vi "1D experiment mouse.vi"() -> ()   [LabVIEW 2011]
uses:
  <vilib>/Platform/TimedLoop/XDataNode/timing_clust.ctl
  <vilib>/Platform/TimedLoop/XDataNode/nitl_modes.ctl
  <vilib>/Platform/TimedLoop/XDataNode/wakeup.ctl
  <vilib>/Utility/inputDevices.llb/closeMouse.vi
  <vilib>/Utility/cursorutil.llb/Set Cursor (Cursor ID).vi
  <vilib>/Utility/inputDevices.llb/mouseAcquire.vi
  <vilib>/Utility/file.llb/Write To Spreadsheet File (DBL).vi
  <vilib>/Utility/file.llb/Write To Spreadsheet File (I64).vi
  <vilib>/Platform/TimedLoop/XDataNode/XDataNode.xnode
  <vilib>/Platform/TimedLoop/XDataNode/XDNodeRunTimeDep.lvlib
  User32.dll
panel:
  out "initial time":u32
  out "1D Experiment":cluster{"Y":dbl[], "Y":dbl[]}[](graph)
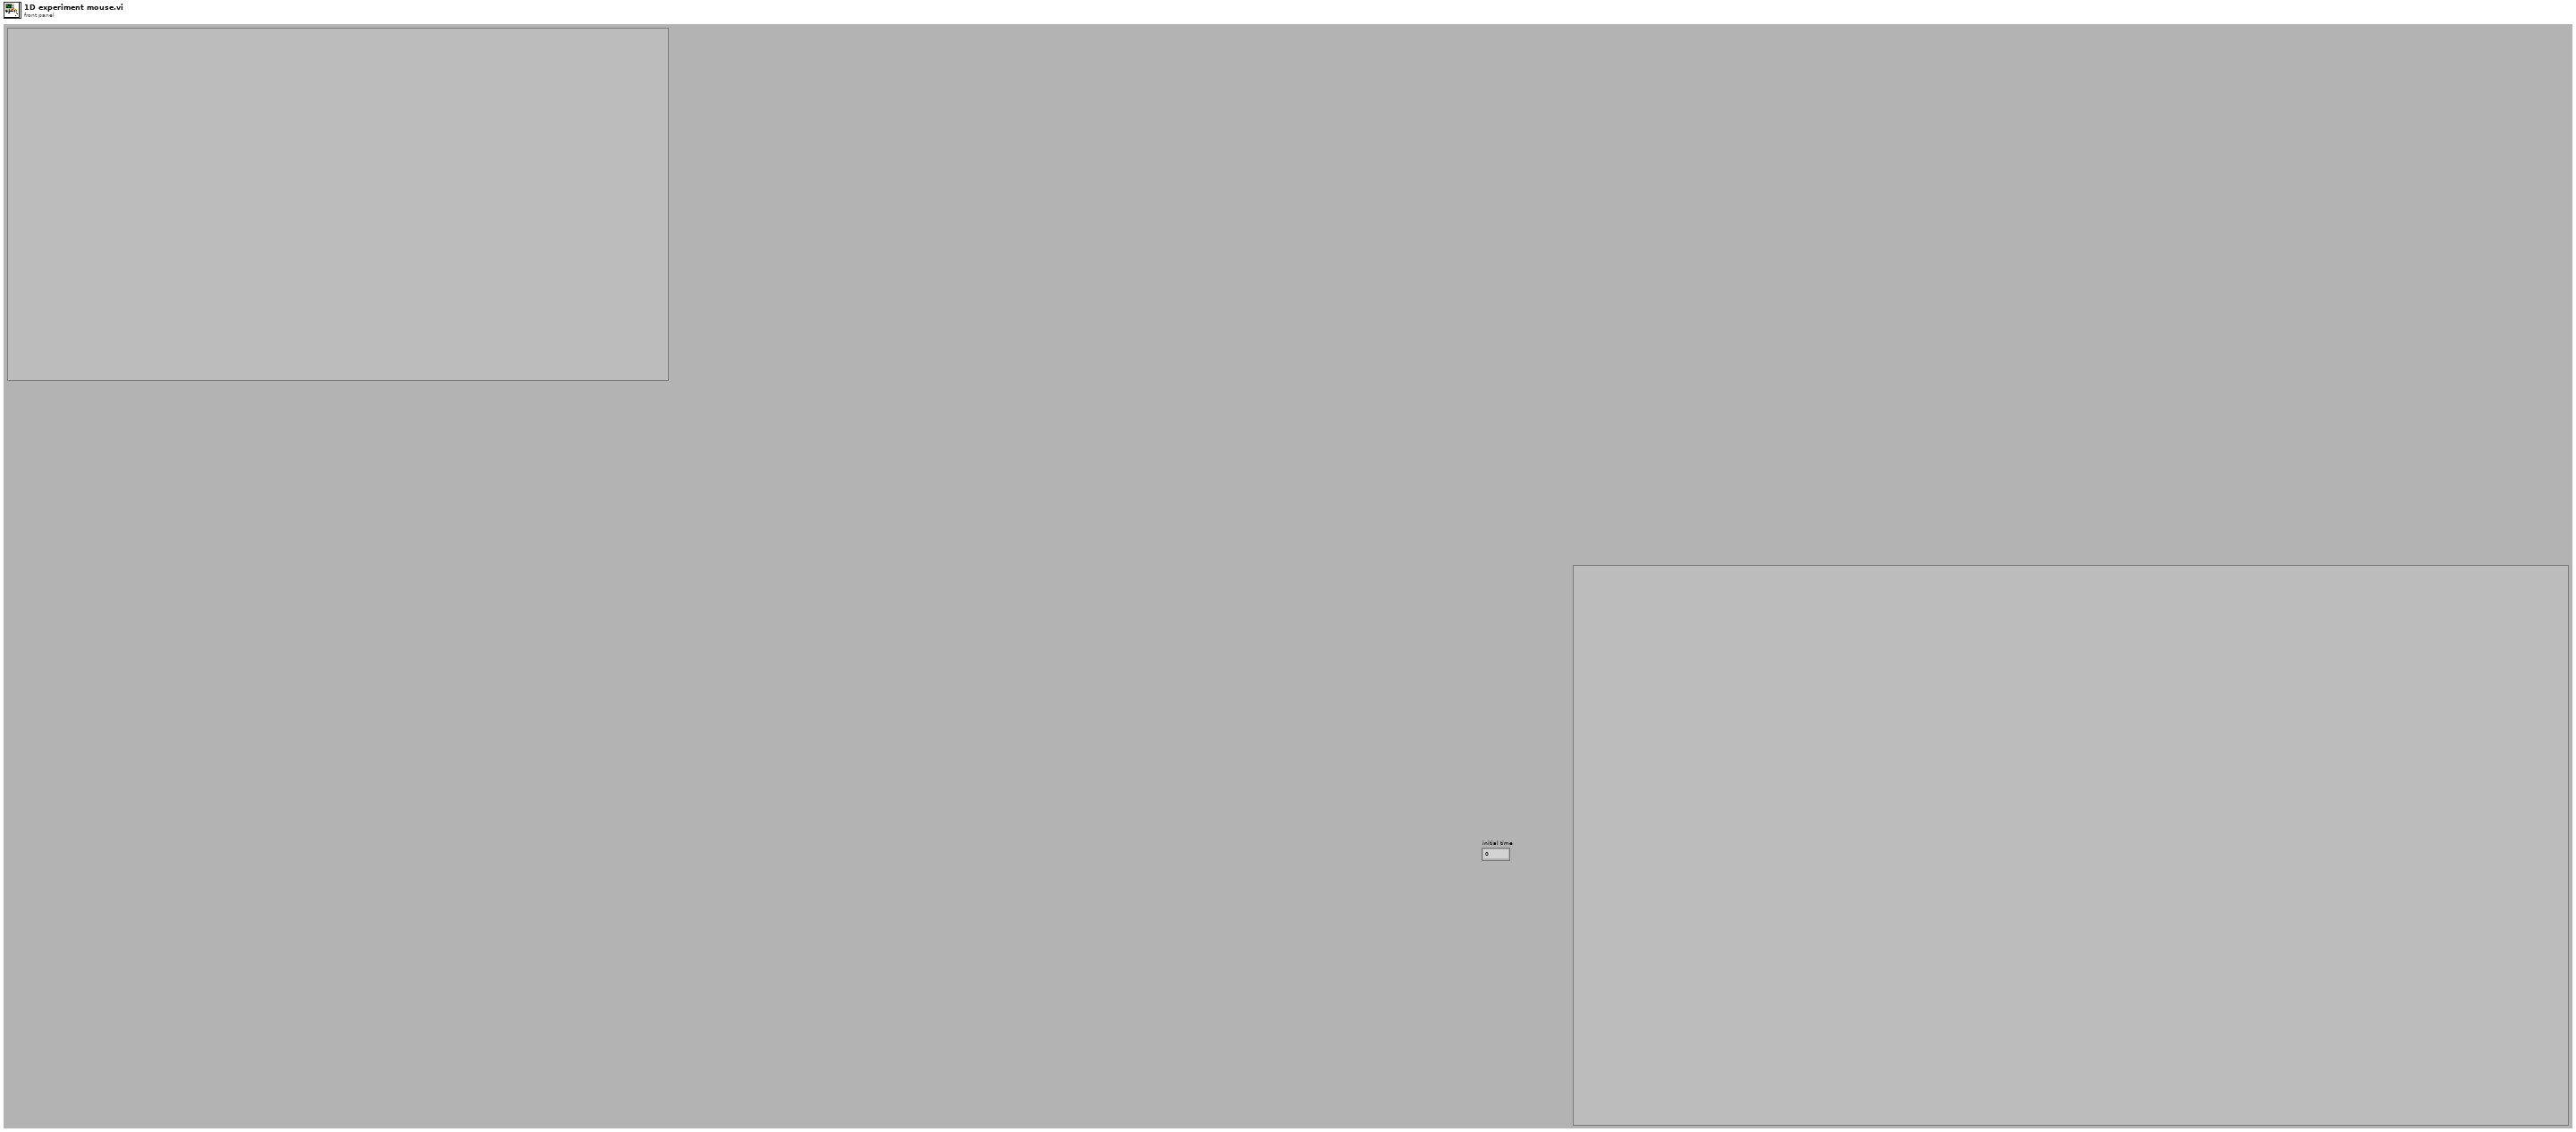
[diagram p1: front panel]
types:
  T1 = enum16{"open", "replace", "create", "open or create", "replace or create", "replace or create with confirmation"}
  T2 = typedef "XDNodeRunTimeDep.lvlib/timing_clust.ctl" = cluster{"Expected End [f-1]":u64, "Actual End [f-1]":u64, "Finished Late? [f-1]":bool, "Expected End [i-1]":u64, "Actual End [i-1]":u64, "Finished Late? [i-1]":bool, "Expected Start [i]":u64, "Actual Start [i]":u64, "Expected Start [f]":u64, "Actual Start [f]":u64, "Source Name":string, "Structure Name":string, "Period":i64, "Deadline":i64, "Offset":i64, "Start":i64, "Priority":i32, "Timeout":i32, "Mode":T3, "Wakeup Reason":T4, "Error":errorcluster, "Source Type":string, "Secondary Source Type":string, "Global End Time":u64, "Global Start Time":u64, "Frame Duration":u64, "Iteration Duration":u64, "Assigned CPU":i32, "I/O Scan Engine Mode":u32}
  T3 = typedef "XDNodeRunTimeDep.lvlib/nitl_modes.ctl" = enum32{"No Change", "Process missed periods, maintain original phase", "Discard missed periods, maintain original phase", "Process missed periods, ignore original phase", "Discard missed periods, ignore original phase"}
  T4 = typedef "XDNodeRunTimeDep.lvlib/wakeup.ctl" = enum32{"Normal", "Aborted", "Asynchronous wakeup", "Timing source error", "Timed loop error", "Timeout"}
  T5 = cluster{"Radius":dbl, "x0":dbl, "y0":dbl, "D":dbl, bool}
  T6 = typedef "LVAllMonitorsDisplayTypeDef.ctl" = cluster{"Bounds":cluster{"Left":i16, "Top":i16, "Right":i16, "Bottom":i16}, "Depth":i16}[]
  T7 = cluster{"Bounds":cluster{"Left":i16, "Top":i16, "Right":i16, "Bottom":i16}, "Depth":i16}
  T8 = cluster{"Left":i16, "Top":i16, "Right":i16, "Bottom":i16}
  T9 = cluster{"Horizontal":i32, "Vertical":i32, "Scrolling":i32}
  T10 = cluster{"button 1":bool, "button 2":bool, "button 3":bool, "button 4":bool}
  T11 = typedef "LVPoint32TypeDef.ctl" = cluster{"Horizontal":i32, "Vertical":i32}
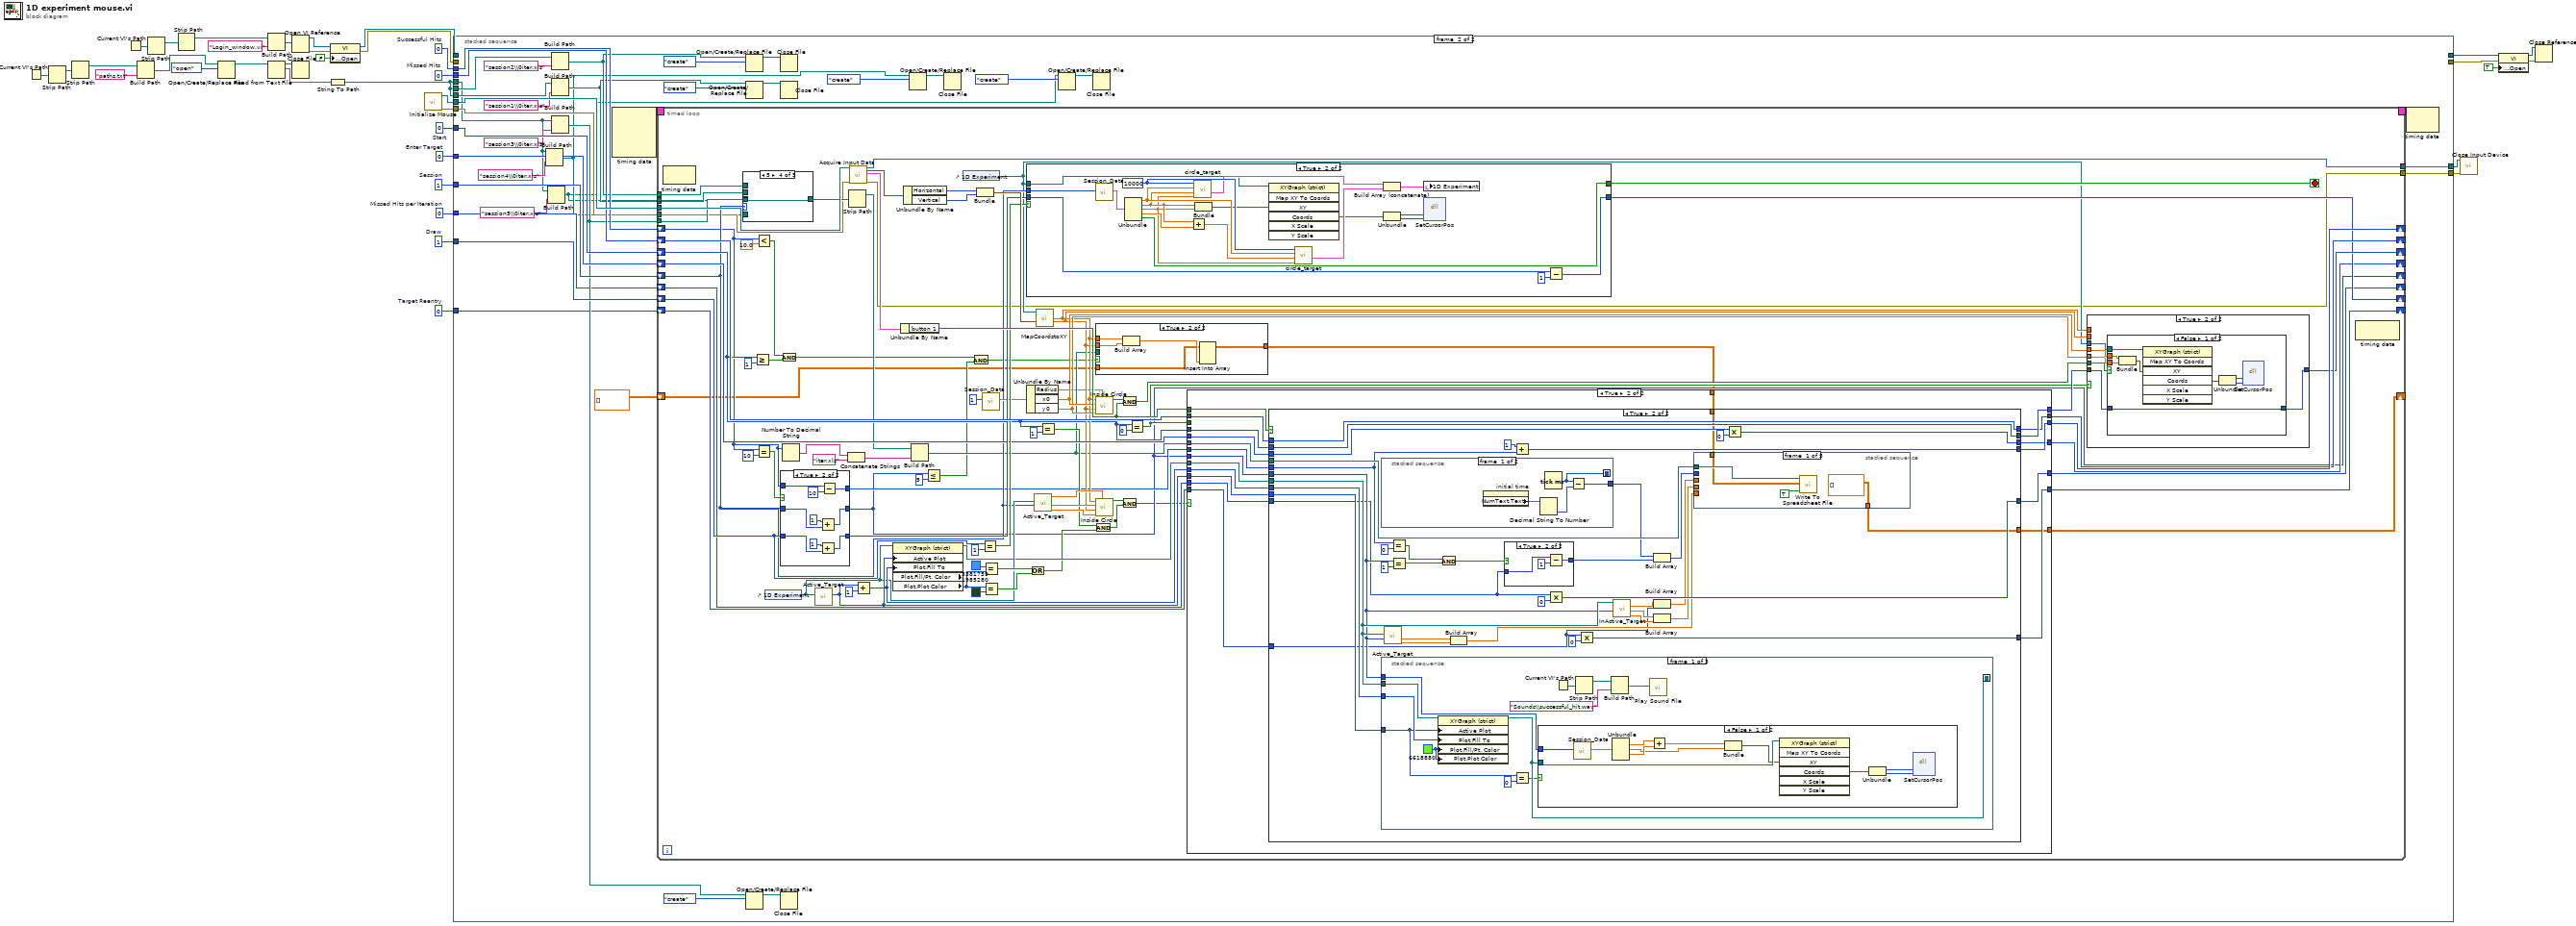
[diagram p0: block diagram]
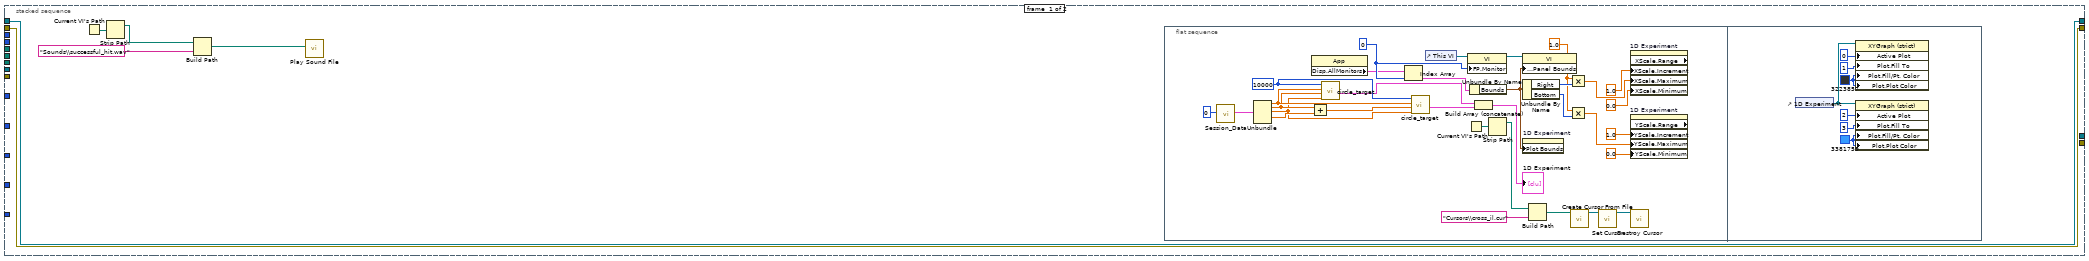
[diagram p2: hidden frame]
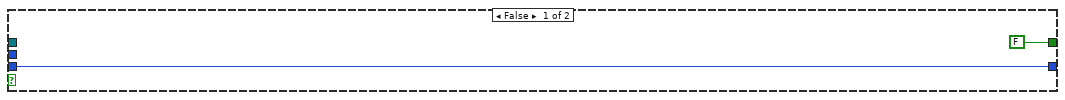
[diagram p8: hidden frame]
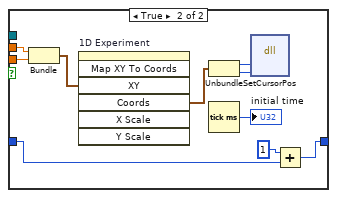
[diagram p10: hidden frame]
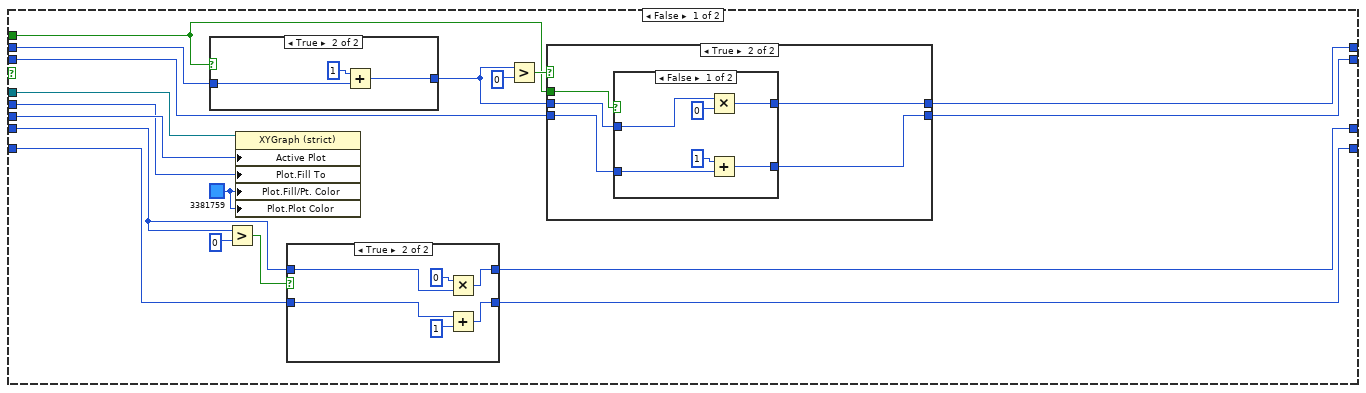
[diagram p13: hidden frame]
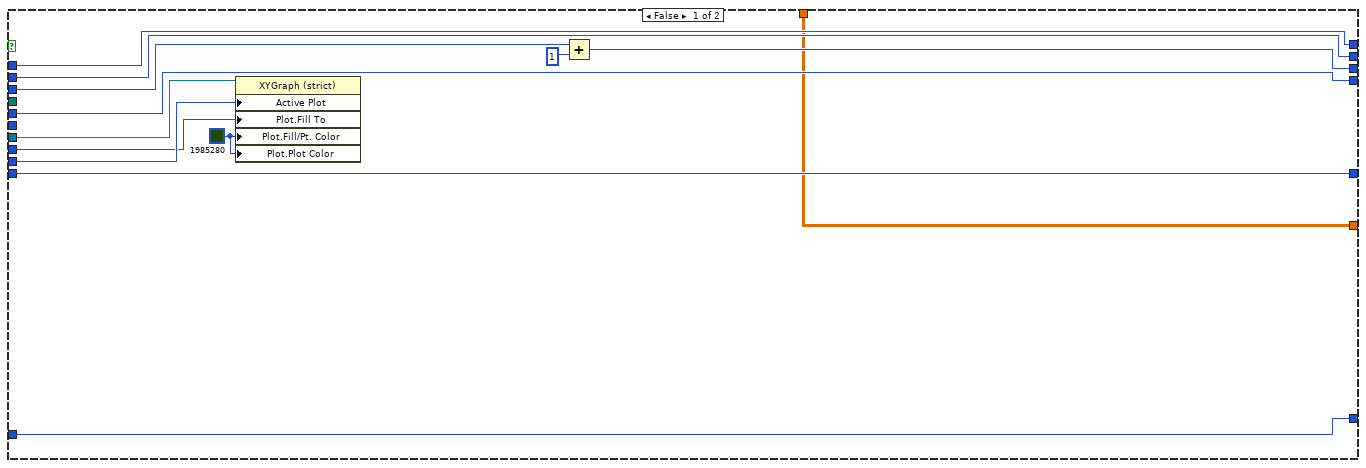
[diagram p18: hidden frame]
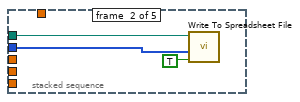
[diagram p20: hidden frame]
diagram:
  w3 = 0  # Target Reentry
  w4 = 0  # Missed Hits per Iteration
  w30 = 0  # Enter Target
  w31 = 1  # Draw
  w32 = 0  # Start
  w33 = 1  # Session
  w34 = 0  # Missed Hits
  w35 = 0  # Successful Hits
  n1 = Current VI's Path() -> (path=w12:path)
  n2 = Strip Path(path=w12) -> (stripped path=w7:path)  [unwired: 1 out]
  n3 = Strip Path(path=w7) -> (stripped path=w8:path)  [unwired: 1 out]
  n4 = Current VI's Path() -> (path=w15:path)
  n5 = Build Path(base path=w8, name or relative path="paths.txt") -> (appended path=w10:path)
  n6 = Strip Path(path=w15) -> (stripped path=w5:path)  [unwired: 1 out]
  n7 = Strip Path(path=w5) -> (stripped path=w6:path)  [unwired: 1 out]
  n8 = Open/Create/Replace File(file path (use dialog)=w10, operation (0:open)=T1."open") -> (refnum out=w28:refnum<file>)  [unwired: 4 in, 2 out]
  n9 = Build Path(base path=w6, name or relative path="Login_window.vi") -> (appended path=w13:path)
  n10 = Read from Text File(file (use dialog)=w28) -> (refnum out=w29:refnum<file>, text=w27:string)  [unwired: 3 in, 2 out]
  n11 = Open VI Reference(vi path=w13) -> (vi reference=w25:refnum<vi>, error out=w24:errorcluster)  [unwired: 5 in]
  n12 = Close File(refnum=w29) -> ()  [unwired: 1 in, 2 out]
  n13 = String To Path(string=w27) -> (path=w26:path)
  n14 = property class="VI"(reference=w25, error in=w24, "Front Panel Window:Open"=FALSE) -> (reference out=w22:refnum<vi>, error out=w21:errorcluster)
  n15 = call <vilib>:"Initialize Mouse.vi"() -> ("error out"=w2:errorcluster, "device ID"=w37:refnum<k1>)  [unwired: 1 in, 9 out]
  n16 = stacked-sequence {
    tunnel: w37 -> [_ w120]
    tunnel: [_ w119] -> w36
    tunnel: w35 -> [_ w118]
    tunnel: w34 -> [_ w117]
    tunnel: w33 -> [_ w113]
    tunnel: w32 -> [_ w116]
    tunnel: w31 -> [_ w115]
    tunnel: w30 -> [_ w114]
    tunnel: w26 -> [_ w103]
    tunnel: w26 -> [_ w110]
    tunnel: w26 -> [_ w90]
    tunnel: w22 -> [w39 _]
    tunnel: w21 -> [w38 _]
    tunnel: [w39 _] -> w17
    tunnel: [w38 _] -> w16
    tunnel: w4 -> [_ w96]
    tunnel: w3 -> [_ w95]
    tunnel: w2 -> [_ w94]
    tunnel: [_ w93] -> w1
    frame #0 {
      n17 = Current VI's Path() -> (path=w41:path)
      n18 = Strip Path(path=w41) -> (stripped path=w40:path)  [unwired: 1 out]
      n19 = Build Path(base path=w40, name or relative path="Sounds\\successful_hit.wav") -> (appended path=w42:path)
      n20 = call <vilib>:"Play Sound File.vi"("path"=w42) -> ()  [unwired: 9 in, 2 out]
      n21 = flat-sequence {
        frame #0 {
          w61 = 1.0 ("y")
          w66 = u16 0 ("Front Panel Window:Monitor")
          w75 = 10000
          n22 = call "Session_Data.vi"("Session"=0) -> ("output cluster"=w53:T5)  [unwired: 10 in]
          n23 = Unbundle(w53) -> ("Radius"=w73:dbl, "x0"=w51:dbl, "y0"=w50:dbl, "D"=w52:dbl)  [unwired: 1 out]
          n24 = Add(x=w51, y=w52) -> (x+y=w74:dbl)
          n25 = property class="App"() -> ("Disp.AllMonitors"=w65:T6)  [unwired: 2 in, 2 out]
          n26 = call "circle_target.vi"("y0"=w50, "x0"=w51, "Radius"=w73, "Pixels"=w75) -> ("Target plots"=w71:cluster{dbl[], dbl[]}[])  [unwired: 7 in]
          n27 = Index Array(array=w65, index=w66) -> (element=w67:T7)
          n28 = call "circle_target.vi"("y0"=w50, "x0"=w74, "Radius"=w73, "Pixels"=w75) -> ("Target plots"=w72:cluster{dbl[], dbl[]}[])  [unwired: 7 in]
          n29 = control-ref of="This VI"() -> (w68:refnum<vi>)
          n30 = Current VI's Path() -> (path=w49:path)
          n31 = property class="VI"(reference=w68, "FP.Monitor"=w66) -> (reference out=w64:refnum<vi>)  [unwired: 1 in, 1 out]
          n32 = Unbundle By Name(w67) -> ("Bounds"=w63:T8)
          n33 = Build Array (concatenate)(w71, w72) -> (→"1D Experiment":cluster{dbl[], dbl[]}[])
          n34 = Strip Path(path=w49) -> (stripped path=w48:path)  [unwired: 1 out]
          n35 = property class="VI"(reference=w64, "Front Panel Window:Panel Bounds"=w63) -> ()  [unwired: 1 in, 2 out]
          n36 = Unbundle By Name(w63) -> ("Right"=w62:i16, "Bottom"=w60:i16)
          n37 = property on="1D Experiment" class="XYGraph (strict)"("Plot Bounds"=w63) -> ()  [unwired: 2 in, 2 out]
          n38 = Build Path(base path=w48, name or relative path="Cursors\\cross_il.cur") -> (appended path=w46:path)
          n39 = Multiply(x=w61, y=w62) -> (x*y=w58:dbl)
          n40 = Multiply(x=w61, y=w60) -> (x*y=w55:dbl)
          n41 = call <vilib>:"Create Cursor From File.vi"("cursor file"=w46) -> ("cursor ID"=w45:refnum<k1>)  [unwired: 9 in, 1 out]
          n42 = call-poly <vilib>:"Set Cursor.vi"("cursor ID"=w45) -> ("previous cursor ID"=w44:refnum<k1>)  [unwired: 9 in, 1 out]
          n43 = property on="1D Experiment" class="XYGraph (strict)" props=["XScale", "Range", "XScale", "Increment", "XScale", "Maximum", "XScale", "Minimum"]("XScale.Increment"=1.0 ("X Scale.Range:Increment"), "XScale.Maximum"=w58, "XScale.Minimum"=0.0 ("X Scale.Range:Minimum")) -> ()  [unwired: 2 in, 3 out]
          n44 = property on="1D Experiment" class="XYGraph (strict)" props=["YScale", "Range", "YScale", "Increment", "YScale", "Maximum", "YScale", "Minimum"]("YScale.Increment"=1.0 ("Y Scale.Range:Increment"), "YScale.Maximum"=w55, "YScale.Minimum"=0.0 ("Y Scale.Range:Minimum")) -> ()  [unwired: 2 in, 3 out]
          n45 = call <vilib>:"Destroy Cursor.vi"("cursor ID"=w44) -> ()  [unwired: 9 in, 1 out]
        }
        frame #1 {
          w81 = u32 3381759
          w78 = u32 3223857
          n46 = control-ref of="1D Experiment"() -> (w82:refnum<vi>)
          n47 = property on="Property Node" class="XYGraph (strict)"(reference=w82, "Active Plot"=u32 0, "Plot.Fill To"=i16 1, "Plot.Fill/Pt. Color"=w78, "Plot.Plot Color"=w78) -> ()  [unwired: 1 in, 2 out]
          n48 = property on="Property Node" class="XYGraph (strict)"(reference=w82, "Active Plot"=u32 2, "Plot.Fill To"=i16 3, "Plot.Fill/Pt. Color"=w81, "Plot.Plot Color"=w81) -> ()  [unwired: 1 in, 2 out]
        }
      }
    }
    frame #1 {
      n49 = Build Path(base path=w90, name or relative path="session4\\0iter.xls") -> (appended path=w85:path)
      n50 = Build Path(base path=w90, name or relative path="session5\\0iter.xls") -> (appended path=w84:path)
      n51 = Build Path(base path=w110, name or relative path="session2\\0iter.xls") -> (appended path=w107:path)
      n52 = Build Path(base path=w103, name or relative path="session1\\0iter.xls") -> (appended path=w99:path)
      n53 = Build Path(base path=w90, name or relative path="session3\\0iter.xls") -> (appended path=w104:path)
      n54 = node-c288() -> (w98:T2)  [unwired: 4 in]
      n55 = timed-loop {
        tunnel: w120 -> [w197]
        tunnel: [w196] -> w119
        shift-right: [w192] -> _
        shift-left: w118 -> [w141]
        shift-right: [w190] -> _
        shift-left: w117 -> [w191]
        shift-right: [w132] -> _
        shift-left: w113 -> [w154]
        shift-right: [w180] -> _
        shift-left: w116 -> [w157]
        shift-right: [w174] -> _
        shift-left: w115 -> [w175]
        shift-right: [w170] -> _
        shift-left: w114 -> [w171]
        tunnel: w99 -> [w155]
        tunnel: w107 -> [w153]
        tunnel: w104 -> [w152]
        timing: w98 -> [_]
        timing-out: [_] -> w97
        shift-right: [w137] -> _
        shift-left: w96 -> [w139]
        shift-right: [w135] -> _
        shift-left: w95 -> [w136]
        tunnel: w94 -> [w127]
        tunnel: [w126] -> w93
        tunnel: w85 -> [w125]
        tunnel: w84 -> [w124]
        shift-right: [w121] -> _
        shift-left: dbl[][] [] -> [w123]
        stop <- w164 stop-if-true
        n56 = node-c288() -> ()  [unwired: 1 in, 1 out]
        n57 = case shown="5" w154 {
          tunnel: w155 -> [_ _ _ _ w214]
          tunnel: [w210 w211 w212 w213 w214] -> w150
          tunnel: w153 -> [w210 _ _ _ _]
          tunnel: w152 -> [_ w211 _ _ _]
          tunnel: w125 -> [_ _ w212 _ _]
          tunnel: w124 -> [_ _ _ w213 _]
          frame 2 {
          }
          frame 3 {
          }
          frame 4 {
          }
          frame 5 {
          }
          frame 1, Default {
          }
        }
        n58 = Greater Or Equal?(x=w157, y=1) -> (x >= y?=w144:bool)
        n59 = Less?(x=w141, y=10.0) -> (x < y?=w143:bool)
        n60 = Equal?(x=w141, y=10) -> (x = y?=w188:bool)
        n61 = control-ref of="1D Experiment"() -> (w186:refnum<vi>)
        n62 = case shown="True" w188 {
          tunnel: w141 -> [w270 w279]
          tunnel: [w270 w277] -> w151
          tunnel: w154 -> [w269 w271]
          tunnel: [w269 w272] -> w132
          tunnel: w175 -> [w268 w275]
          tunnel: [w268 w273] -> w173
          frame False {
          }
          frame True {
            n63 = Add(x=1, y=w271) -> (x+y=w272:i32)
            n64 = Add(x=1, y=w275) -> (x+y=w273:i32)
            n65 = Subtract(x=w279, y=10) -> (x-y=w277:i32)
          }
        }
        n66 = And(x=w143, y=w144) -> (x .and. y?=w133:bool)
        n67 = Number To Decimal String(number=w141) -> (decimal integer string=w149:string)  [unwired: 1 in]
        n68 = call "Active_Target.vi"("XYGraph Refnum"=w186) -> ("Active Plot"=w202:u32)  [unwired: 7 in, 3 out]
        n69 = Concatenate Strings(w149, "iter.xls" ("name or relative path")) -> (w147:string)
        n70 = Strip Path(path=w150) -> (stripped path=w146:path)  [unwired: 1 out]
        n71 = call-poly <vilib>:"Acquire Input Data.vi"("device ID"=w197, "error in (no error)"=w127) -> ("device ID"=w196:refnum<k1>, "axis info"=w195:T9, "button info"=w198:T10, "error out"=w126:errorcluster)  [unwired: 1 in, 13 out]
        n72 = Add(x=w202, y=u32 1) -> (x+y=w201:u32)
        n73 = property on="Property Node" class="XYGraph (strict)" props=["Active Plot", "Plot", "Fill To", "Plot", "Fill/Pt. Color", "Plot", "Plot Color"](reference=w186, "Active Plot"=w202, "Plot.Fill To"=w201) -> (reference out=w177:refnum<vi>, "Plot.Plot Color"=w179:u32)  [unwired: 1 in, 2 out]
        n74 = Unbundle By Name(w198) -> ("button 1"=w183:bool)
        n75 = Unbundle By Name(w195) -> ("Horizontal"=w194:i32, "Vertical"=w193:i32)
        n76 = Build Path(base path=w146, name or relative path=w147) -> (appended path=w145:path)
        n77 = Less Or Equal?(x=w132, y=5) -> (x <= y?=w129:bool)
        n78 = control-ref of="1D Experiment"() -> (w140:refnum<vi>)
        n79 = And(x=w133, y=w129) -> (x .and. y?=w130:bool)
        n80 = Bundle("Horizontal"=w194, "Vertical"=w193) -> (w184:cluster{"Horizontal":i32, "Vertical":i32})  [unwired: 1 in]
        n81 = Equal?(x=w175, y=1) -> (x = y?=w172:bool)
        n82 = call "Session_Data.vi"("Session"=1) -> ("output cluster"=w163:T5)  [unwired: 10 in]
        n83 = Equal?(x=u32 3381759, y=w179) -> (x = y?=w205:bool)
        n84 = Equal?(x=w179, y=u32 1985280) -> (x = y?=w204:bool)
        n85 = case shown="True" w172 {
          tunnel: w154 -> [_ w231]
          tunnel: [w221 w241] -> w174
          tunnel: w173 -> [w221 w240]
          tunnel: [FALSE ("Valid") w230] -> w164
          tunnel: w140 -> [_ w226]
          frame False {
          }
          frame True {
            w239 = 10000
            n86 = call "Session_Data.vi"("Session"=w231) -> ("output cluster"=w234:T5)  [unwired: 10 in]
            n87 = Unbundle(w234) -> ("Radius"=w237:dbl, "x0"=w225:dbl, "y0"=w224:dbl, "D"=w233:dbl, w230:bool)
            n88 = Add(x=w225, y=w233) -> (x+y=w238:dbl)
            n89 = call "circle_target.vi"("y0"=w224, "x0"=w225, "Radius"=w237, "Pixels"=w239) -> ("Target plots"=w235:cluster{dbl[], dbl[]}[])  [unwired: 7 in]
            n90 = Bundle("x0"=w225, "y0"=w224) -> (w223:cluster{"x0":dbl, "y0":dbl})  [unwired: 1 in]
            n91 = invoke on="Invoke Node" class="XYGraph (strict)" method="Map XY To Coords"(reference=w226, "XY"=w223) -> ("Coords"=w229:T11)  [unwired: 5 in, 6 out]
            n92 = call "circle_target.vi"("y0"=w224, "x0"=w238, "Radius"=w237, "Pixels"=w239) -> ("Target plots"=w236:cluster{dbl[], dbl[]}[])  [unwired: 7 in]
            n93 = Build Array (concatenate)(w235, w236) -> (w232:cluster{dbl[], dbl[]}[])
            n94 = Unbundle(w229) -> ("Horizontal"=w228:i32, "Vertical"=w227:i32)
            n95 = local write "1D Experiment"(w232) -> ()
            n96 = dll-call lib="User32.dll" fn="SetCursorPos"(w228, w227) -> ()  [unwired: 6 in, 2 out]
            n97 = Subtract(x=w240, y=1) -> (x-y=w241:i32)
          }
        }
        n98 = Unbundle By Name(w163) -> ("Radius"=w134:dbl, "x0"=w162:dbl, "y0"=w161:dbl)
        n99 = Or(x=w205, y=w204) -> (x .or. y?=w168:bool)
        n100 = call "Active_Target.vi"("Session"=w154, "XYGraph Refnum"=w186) -> ("y0"=w199:dbl, "x0"=w200:dbl, "Radius"=w187:dbl)  [unwired: 6 in, 1 out]
        n101 = call "MapCoordstoXY.vi"("Coordinates"=w184, "XYGraph Refnum"=w140) -> ("Y(graph)"=w158:dbl, "X (graph)"=w159:dbl)  [unwired: 7 in]
        n102 = Equal?(x=w157, y=1) -> (x = y?=w166:bool)
        n103 = And(x=w166, y=w168) -> (x .and. y?=w165:bool)
        n104 = case shown="True" w130 {
          tunnel: w159 -> [_ w220]
          tunnel: w158 -> [_ w219]
          tunnel: w145 -> [_ _]
          tunnel: w123 -> [w215 w217]
          tunnel: [w215 w216] -> w122
          frame False {
          }
          frame True {
            n105 = Build Array(w220, w219) -> (w218:dbl[])
            n106 = Insert Into Array(array=w217, new element=w218) -> (w216:dbl[][])  [unwired: 2 in]
          }
        }
        n107 = call "Inside Circle.vi"("Radius"=w134, "y0"=w161, "y"=w158, "x0"=w162, "x"=w159) -> ("Inside Circle"=w182:bool)  [unwired: 6 in]
        n108 = call "Inside Circle.vi"("Radius"=w187, "y0"=w199, "y"=w158, "x0"=w200, "x"=w159) -> ("Inside Circle"=w167:bool)  [unwired: 6 in]
        n109 = And(x=w182, y=w183) -> (x .and. y?=w181:bool)
        n110 = And(x=w167, y=w165) -> (x .and. y?=w128:bool)
        n111 = Equal?(x=w157, y=0) -> (x = y?=w138:bool)
        n112 = case shown="True" w128 {
          tunnel: w183 -> [w289 w364]
          tunnel: w202 -> [w293 w361]
          tunnel: w201 -> [w292 w360]
          tunnel: w151 -> [w295 w363]
          tunnel: [w295 w362] -> w192
          tunnel: w191 -> [w294 w352]
          tunnel: [w286 w350] -> w190
          tunnel: w157 -> [w291 w359]
          tunnel: [w291 w358] -> w178
          tunnel: w177 -> [w290 w357]
          tunnel: w171 -> [w284 w356]
          tunnel: [w283 w355] -> w170
          tunnel: w132 -> [_ w354]
          tunnel: w145 -> [_ w353]
          tunnel: w139 -> [w288 w351]
          tunnel: w138 -> [w287 _]
          tunnel: [w285 w349] -> w137
          tunnel: w136 -> [w282 w348]
          tunnel: [w281 w347] -> w135
          tunnel: w122 -> [w280 w346]
          tunnel: [w280 w345] -> w121
          frame False {
            n113 = case shown="True" w287 {
              tunnel: w294 -> [w312 w343]
              tunnel: w293 -> [w311 _]
              tunnel: w292 -> [w310 _]
              tunnel: w290 -> [w309 _]
              tunnel: w289 -> [w306 _]
              tunnel: w288 -> [w304 w344]
              tunnel: [w303 w343] -> w286
              tunnel: [w302 w344] -> w285
              tunnel: w284 -> [w299 w342]
              tunnel: [w298 w342] -> w283
              tunnel: w282 -> [w297 w341]
              tunnel: [w296 w341] -> w281
              frame False {
                w313 = u32 3381759
                n114 = case shown="True" w306 {
                  tunnel: w312 -> [w337 w340]
                  tunnel: [w337 w338] -> w305
                  frame False {
                  }
                  frame True {
                    n115 = Add(x=1, y=w340) -> (x+y=w338:i32)
                  }
                }
                n116 = Greater?(x=w299, y=0) -> (0:w300:bool)
                n117 = property on="Property Node" class="XYGraph (strict)"(reference=w309, "Active Plot"=w311, "Plot.Fill To"=w310, "Plot.Fill/Pt. Color"=w313, "Plot.Plot Color"=w313) -> ()  [unwired: 1 in, 2 out]
                n118 = case shown="True" w300 {
                  tunnel: w299 -> [w315 w321]
                  tunnel: [w315 w319] -> w298
                  tunnel: w297 -> [w314 w318]
                  tunnel: [w314 w316] -> w296
                  frame False {
                  }
                  frame True {
                    n119 = Multiply(x=0, y=w321) -> (x*y=w319:i32)
                    n120 = Add(x=w318, y=1) -> (x+y=w316:i32)
                  }
                }
                n121 = Greater?(x=w305, y=0) -> (0:w307:bool)
                n122 = case shown="True" w307 {
                  tunnel: [w322 w328] -> w302
                  tunnel: [w323 w327] -> w303
                  tunnel: w306 -> [_ w326]
                  tunnel: w305 -> [w323 w325]
                  tunnel: w304 -> [w322 w324]
                  frame False {
                  }
                  frame True {
                    n123 = case shown="False" w326 {
                      tunnel: [w333 w336] -> w328
                      tunnel: [w331 w335] -> w327
                      tunnel: w325 -> [w330 w335]
                      tunnel: w324 -> [w329 w336]
                      frame False {
                        n124 = Multiply(x=w330, y=0) -> (x*y=w331:i32)
                        n125 = Add(x=1, y=w329) -> (x+y=w333:i32)
                      }
                      frame True {
                      }
                    }
                  }
                }
              }
              frame True {
              }
            }
          }
          frame True {
            n126 = case shown="True" w364 {
              tunnel: w363 -> [w376 w390]
              tunnel: [w376 w410] -> w362
              tunnel: w361 -> [w375 w413]
              tunnel: w360 -> [w374 w412]
              tunnel: w359 -> [w372 w411]
              tunnel: [w372 w411] -> w358
              tunnel: w357 -> [w373 w397]
              tunnel: w356 -> [w368 w402]
              tunnel: [w369 w400] -> w355
              tunnel: w354 -> [_ w388]
              tunnel: w353 -> [_ w408]
              tunnel: w352 -> [w371 w406]
              tunnel: [w371 w406] -> w350
              tunnel: w351 -> [w370 w383]
              tunnel: [w370 w404] -> w349
              tunnel: w348 -> [w366 w381]
              tunnel: [w366 w399] -> w347
              tunnel: w346 -> [w365 w379]
              tunnel: [w365 w378] -> w345
              frame False {
                w377 = u32 1985280
                n127 = property on="Property Node" class="XYGraph (strict)"(reference=w373, "Active Plot"=w375, "Plot.Fill To"=w374, "Plot.Fill/Pt. Color"=w377, "Plot.Plot Color"=w377) -> ()  [unwired: 1 in, 2 out]
                n128 = Add(x=w368, y=1) -> (x+y=w369:i32)
              }
              frame True {
                n129 = stacked-sequence {
                  seq-local: [w435 _] -> [_ w439]
                  tunnel: [w436 _] -> w407
                  frame #0 {
                    n130 = property on="initial time" class="DigNum (strict)"() -> ("NumText.Text"=w438:string)  [unwired: 2 in, 2 out]
                    n131 = Decimal String To Number(string=w438) -> (number=w437:i32)  [unwired: 2 in, 1 out]
                    n132 = Tick Count (ms)() -> (millisecond timer value=w435:u32)
                    n133 = Subtract(x=w435, y=w437) -> (x-y=w436:u32)
                  }
                  frame #1 {
                    n134 = Number To Decimal String(number=w439) -> (decimal integer string=w440:string)  [unwired: 1 in]
                    n135 = property on="initial time" class="DigNum (strict)"("NumText.Text"=w440) -> ()  [unwired: 2 in, 2 out]
                  }
                }
                n136 = stacked-sequence {
                  seq-local: [w449 _ _] -> [_ w473 w482]
                  tunnel: w413 -> [w448 w474 w484]
                  tunnel: w412 -> [w451 _ w483]
                  tunnel: w397 -> [w450 _ _]
                  tunnel: w388 -> [w445 _ _]
                  frame #0 {
                    w452 = u32 6618880
                    n137 = property on="Property Node" class="XYGraph (strict)"(reference=w450, "Active Plot"=w448, "Plot.Fill To"=w451, "Plot.Fill/Pt. Color"=w452, "Plot.Plot Color"=w452) -> (reference out=w449:refnum<vi>)  [unwired: 1 in, 1 out]
                    n138 = Equal?(x=w448, y=u32 0) -> (x = y?=w446:bool)
                    n139 = case shown="False" w446 {
                      tunnel: w449 -> [w459 w465]
                      tunnel: w445 -> [w457 w469]
                      frame False {
                        n140 = call "Session_Data.vi"("Session"=w457) -> ("output cluster"=w460:T5)  [unwired: 10 in]
                        n141 = Unbundle(w460) -> ("x0"=w455:dbl, "y0"=w453:dbl, "D"=w454:dbl)  [unwired: 2 out]
                        n142 = Add(x=w455, y=w454) -> (x+y=w456:dbl)
                        n143 = Bundle(w456, "y0"=w453) -> (w458:cluster{dbl, "y0":dbl})  [unwired: 1 in]
                        n144 = invoke on="Invoke Node" class="XYGraph (strict)" method="Map XY To Coords"(reference=w459, "XY"=w458) -> ("Coords"=w463:T11)  [unwired: 5 in, 6 out]
                        n145 = Unbundle(w463) -> ("Horizontal"=w462:i32, "Vertical"=w461:i32)
                        n146 = dll-call lib="User32.dll" fn="SetCursorPos"(w462, w461) -> ()  [unwired: 6 in, 2 out]
                      }
                      frame True {
                        n147 = call "Session_Data.vi"("Session"=w469) -> ("output cluster"=w468:T5)  [unwired: 10 in]
                        n148 = Unbundle(w468) -> ("x0"=w467:dbl, "y0"=w464:dbl)  [unwired: 3 out]
                        n149 = Bundle("x0"=w467, "y0"=w464) -> (w466:cluster{"x0":dbl, "y0":dbl})  [unwired: 1 in]
                        n150 = invoke on="Invoke Node" class="XYGraph (strict)" method="Map XY To Coords"(reference=w465, "XY"=w466) -> ("Coords"=w472:T11)  [unwired: 5 in, 6 out]
                        n151 = Unbundle(w472) -> ("Horizontal"=w471:i32, "Vertical"=w470:i32)
                        n152 = dll-call lib="User32.dll" fn="SetCursorPos"(w471, w470) -> ()  [unwired: 6 in, 2 out]
                      }
                    }
                    n153 = Current VI's Path() -> (path=w442:path)
                    n154 = Strip Path(path=w442) -> (stripped path=w441:path)  [unwired: 1 out]
                    n155 = Build Path(base path=w441, name or relative path="Sounds\\successful_hit.wav") -> (appended path=w443:path)
                    n156 = call <vilib>:"Play Sound File.vi"("path"=w443) -> ()  [unwired: 9 in, 2 out]
                  }
                  frame #1 {
                    w481 = u32 3381759
                    n157 = Subtract(x=w474, y=u32 2) -> (x-y=w478:u32)
                    n158 = To Long Integer(number=w478) -> (32bit integer=w477:i32)
                    n159 = Absolute Value(x=w477) -> (abs(x)=w475:i32)
                    n160 = Add(x=w475, y=u32 1) -> (x+y=w479:u32)
                    n161 = property on="Property Node" class="XYGraph (strict)"(reference=w473, "Active Plot"=w475, "Plot.Fill To"=w479, "Plot.Fill/Pt. Color"=w481, "Plot.Plot Color"=w481) -> ()  [unwired: 1 in, 2 out]
                  }
                  frame #2 {
                    w485 = u32 3223857
                    n162 = property on="Property Node" class="XYGraph (strict)"(reference=w482, "Active Plot"=w484, "Plot.Fill To"=w483, "Plot.Fill/Pt. Color"=w485, "Plot.Plot Color"=w485) -> ()  [unwired: 1 in, 2 out]
                  }
                }
                n163 = call "Active_Target.vi"("Session"=w388, "XYGraph Refnum"=w397) -> ("y0"=w392:dbl, "x0"=w393:dbl)  [unwired: 6 in, 2 out]
                n164 = Equal?(x=w390, y=0) -> (x = y?=w386:bool)
                n165 = Equal?(x=w388, y=1) -> (x = y?=w385:bool)
                n166 = And(x=w386, y=w385) -> (x .and. y?=w384:bool)
                n167 = Build Array(w393, w392) -> (w391:dbl[])
                n168 = case shown="True" w384 {
                  tunnel: w383 -> [w415 w418]
                  tunnel: [w415 w416] -> w382
                  frame False {
                  }
                  frame True {
                    n169 = Subtract(x=w418, y=1) -> (x-y=w416:i32)
                  }
                }
                n170 = Add(x=1, y=w390) -> (x+y=w410:i32)
                n171 = Multiply(x=w383, y=0) -> (x*y=w404:i32)
                n172 = Multiply(x=w381, y=0) -> (x*y=w399:i32)
                n173 = call "InActive_Target.vi"("Session"=w388, "XYGraph Refnum"=w397) -> ("y0"=w395:dbl, "x0"=w396:dbl, "Radius"=w380:dbl)  [unwired: 5 in, 1 out]
                n174 = Build Array(w407, w382) -> (w409:u32[])
                n175 = Build Array(w380, w381) -> (w398:dbl[])
                n176 = Build Array(w396, w395) -> (w394:dbl[])
                n177 = stacked-sequence {
                  tunnel: w409 -> [_ w425 _ _ _]
                  tunnel: w408 -> [w421 w423 w428 w431 w434]
                  tunnel: w398 -> [_ _ w427 _ _]
                  tunnel: w394 -> [_ _ _ w429 _]
                  tunnel: w391 -> [_ _ _ _ w432]
                  tunnel: w379 -> [w420 _ _ _ _]
                  tunnel: [dbl[][] [] _ _ _ _] -> w378
                  frame #0 {
                    n178 = call-poly <vilib>:"Write To Spreadsheet File.vi"("append to file? (new file:F)"=TRUE, "2D data"=w420, "file path (dialog if empty)"=w421) -> ()  [unwired: 5 in, 1 out]
                  }
                  frame #1 {
                    n179 = call-poly <vilib>:"Write To Spreadsheet File.vi"("append to file? (new file:F)"=TRUE, "1D data"=w425, "file path (dialog if empty)"=w423) -> ()  [unwired: 5 in, 1 out]
                  }
                  frame #2 {
                    n180 = call-poly <vilib>:"Write To Spreadsheet File.vi"("append to file? (new file:F)"=TRUE, "1D data"=w427, "file path (dialog if empty)"=w428) -> ()  [unwired: 5 in, 1 out]
                  }
                  frame #3 {
                    n181 = call-poly <vilib>:"Write To Spreadsheet File.vi"("append to file? (new file:F)"=TRUE, "1D data"=w429, "file path (dialog if empty)"=w431) -> ()  [unwired: 5 in, 1 out]
                  }
                  frame #4 {
                    n182 = call-poly <vilib>:"Write To Spreadsheet File.vi"("append to file? (new file:F)"=TRUE, "1D data"=w432, "file path (dialog if empty)"=w434) -> ()  [unwired: 5 in, 1 out]
                  }
                }
                n183 = Multiply(x=w402, y=0) -> (x*y=w400:i32)
              }
            }
          }
        }
        n184 = case shown="True" w138 {
          tunnel: w140 -> [_ w244]
          tunnel: w159 -> [_ _]
          tunnel: w158 -> [_ _]
          tunnel: w181 -> [_ w249]
          tunnel: w178 -> [w243 w248]
          tunnel: [w243 w247] -> w180
          tunnel: w162 -> [_ w246]
          tunnel: w161 -> [_ w245]
          frame False {
          }
          frame True {
            n185 = case shown="False" w249 {
              tunnel: w248 -> [w257 w267]
              tunnel: [w257 w265] -> w247
              tunnel: w246 -> [w256 w260]
              tunnel: w245 -> [w255 w259]
              tunnel: w244 -> [w250 _]
              frame False {
                n186 = Bundle("x0"=w256, "y0"=w255) -> (w254:cluster{"x0":dbl, "y0":dbl})  [unwired: 1 in]
                n187 = invoke on="Invoke Node" class="XYGraph (strict)" method="Map XY To Coords"(reference=w250, "XY"=w254) -> ("Coords"=w251:T11)  [unwired: 5 in, 6 out]
                n188 = Unbundle(w251) -> ("Horizontal"=w253:i32, "Vertical"=w252:i32)
                n189 = dll-call lib="User32.dll" fn="SetCursorPos"(w253, w252) -> ()  [unwired: 6 in, 2 out]
              }
              frame True {
                n190 = Bundle("x0"=w260, "y0"=w259) -> (w264:cluster{"x0":dbl, "y0":dbl})  [unwired: 1 in]
                n191 = invoke on="1D Experiment" class="XYGraph (strict)" method="Map XY To Coords"("XY"=w264) -> ("Coords"=w263:T11)  [unwired: 6 in, 6 out]
                n192 = Unbundle(w263) -> ("Horizontal"=w262:i32, "Vertical"=w261:i32)
                n193 = Tick Count (ms)() -> (millisecond timer value=→"initial time":u32)
                n194 = dll-call lib="User32.dll" fn="SetCursorPos"(w262, w261) -> ()  [unwired: 6 in, 2 out]
                n195 = Add(x=1, y=w267) -> (x+y=w265:i32)
              }
            }
          }
        }
        n196 = node-c288() -> ()  [unwired: 1 in, 1 out]
      }
      n197 = Open/Create/Replace File(file path (use dialog)=w107, operation (0:open)=T1."create") -> (refnum out=w109:refnum<file>)  [unwired: 4 in, 2 out]
      n198 = Open/Create/Replace File(file path (use dialog)=w99, operation (0:open)=T1."create") -> (refnum out=w101:refnum<file>)  [unwired: 4 in, 2 out]
      n199 = Open/Create/Replace File(file path (use dialog)=w104, operation (0:open)=T1."create") -> (refnum out=w106:refnum<file>)  [unwired: 4 in, 2 out]
      n200 = Close File(refnum=w109) -> ()  [unwired: 1 in, 2 out]
      n201 = Close File(refnum=w101) -> ()  [unwired: 1 in, 2 out]
      n202 = Close File(refnum=w106) -> ()  [unwired: 1 in, 2 out]
      n203 = Open/Create/Replace File(file path (use dialog)=w85, operation (0:open)=T1."create") -> (refnum out=w89:refnum<file>)  [unwired: 4 in, 2 out]
      n204 = Close File(refnum=w89) -> ()  [unwired: 1 in, 2 out]
      n205 = Open/Create/Replace File(file path (use dialog)=w84, operation (0:open)=T1."create") -> (refnum out=w87:refnum<file>)  [unwired: 4 in, 2 out]
      n206 = Close File(refnum=w87) -> ()  [unwired: 1 in, 2 out]
      n207 = node-c288(w97) -> ()  [unwired: 1 out]
    }
  }
  n208 = call-poly <vilib>:"Close Input Device.vi"("error in (no error)"=w1, "device ID"=w36) -> ()  [unwired: 9 out]
  n209 = property class="VI"(reference=w17, error in=w16, "Front Panel Window:Open"=TRUE) -> (reference out=w19:refnum<vi>, error out=w18:errorcluster)
  n210 = Close Reference(reference=w19, error in (no error)=w18) -> ()  [unwired: 1 out]
